vi "Register gRPC Messages.vi"(8 "error in (no error)":errorcluster, 11 "gRPC ID":T1) -> (0 "error out":errorcluster, 3 "gRPC ID Out":T1)   [LabVIEW 2019, in "Generated_server.lvlib"]
uses:
  Generated_server.lvlib
  <vilib>/gRPC/LabVIEW gRPC Library/grpc-lvsupport-release.lvlib
  <vilib>/gRPC/LabVIEW gRPC Library/Server API/typeDefs/Message Metadata.ctl
  <vilib>/gRPC/LabVIEW gRPC Library/Server API/typeDefs/Message Element Type.ctl
  <vilib>/gRPC/LabVIEW gRPC Library/Server API/typeDefs/Message Element Metadata.ctl
  <vilib>/gRPC/LabVIEW gRPC Library/Server API/typeDefs/Enum Metadata.ctl
  <vilib>/gRPC/LabVIEW gRPC Library/Shared/grpcId.ctl
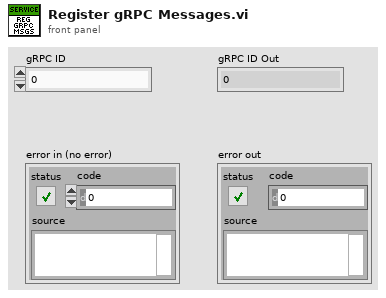
[diagram p1: front panel]
types:
  T1 = typedef "grpc-lvsupport-release.lvlib/grpcId.ctl" = u64
  T2 = typedef "grpc-lvsupport-release.lvlib/Enum Metadata.ctl" = cluster{"Version":i32, "Name":string, "Type Url":string, "Enum Values":string, "Allow Alias":bool}
  T3 = typedef "grpc-lvsupport-release.lvlib/Message Metadata.ctl" = cluster{"Version":i32, "Name":string, "Type Url":string, "Elements":T4[], "Has Oneof":bool}
  T4 = typedef "grpc-lvsupport-release.lvlib/Message Element Metadata.ctl" = cluster{"Field Name":string, "Embedded Message Name":string, "Protobuf Index":i32, "MessageElementType":T5, "Repeated":bool, "Is in Oneof":bool, "Oneof Container Name":string}
  T5 = typedef "grpc-lvsupport-release.lvlib/Message Element Type.ctl" = enum32{"Int32Value", "FloatValue", "DoubleValue", "BoolValue", "StringValue", "MessageValue", "Int64Value", "UInt32Value", "UInt64Value", "EnumValue", "Bytes", "Fixed64", "Fixed32", "SFixed64", "SFixed32", "SInt64", "SInt32"}
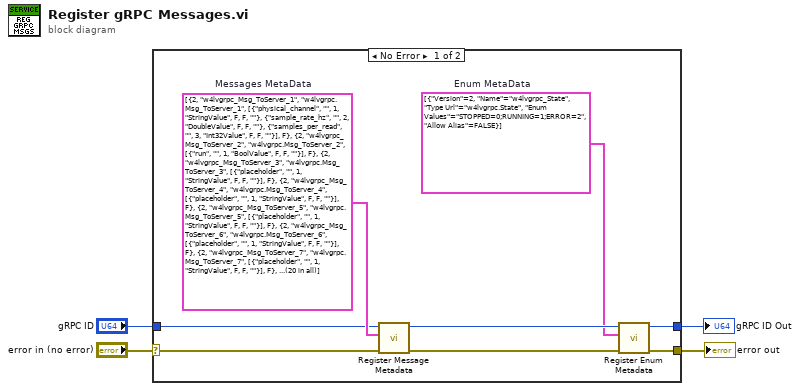
[diagram p0: block diagram]
diagram:
  n1 = case shown="No Error" "error in (no error)" {
    selector: "error in (no error)" -> [w10 w13]
    tunnel: [w9 w12] -> w2
    tunnel: [w6 w13] -> w1
    tunnel: "gRPC ID" -> [w9 w12]
    frame No Error {
      w5 = T2[] [{"Version"=2, "Name"="w4lvgrpc_State", "Type Url"="w4lvgrpc.State", "Enum Values"="STOPPED=0;RUNNING=1;ERROR=2", "Allow Alias"=FALSE}]  # Enum MetaData
      w11 = T3[] [{"Version"=2, "Name"="w4lvgrpc_Msg_ToServer_1", "Type Url"="w4lvgrpc.Msg_ToServer_1", "Elements"=[{"Field Name"="physical_channel", "Embedded Message Name"="", "Protobuf Index"=1, "MessageElementType"=enum."StringValue", "Repeated"=FALSE, "Is in Oneof"=FALSE, "Oneof Container Name"=""}, {"Field Name"="sample_rate_hz", "Embedded Message Name"="", "Protobuf Index"=2, "MessageElementType"=enum."DoubleValue", "Repeated"=FALSE, "Is in Oneof"=FALSE, "Oneof Container Name"=""}, {"Field Name"="samples_per_read", "Embedded Message Name"="", "Protobuf Index"=3, "MessageElementType"=enum."Int32Value", "Repeated"=FALSE, "Is in Oneof"=FALSE, "Oneof Container Name"=""}], "Has Oneof"=FALSE}, {"Version"=2, "Name"="w4lvgrpc_Msg_ToServer_2", "Type Url"="w4lvgrpc.Msg_ToServer_2", "Elements"=[{"Field Name"="run", "Embedded Message Name"="", "Protobuf Index"=1, "MessageElementType"=enum."BoolValue", "Repeated"=FALSE, "Is in Oneof"=FALSE, "Oneof Container Name"=""}], "Has Oneof"=FALSE}, {"Version"=2, "Name"="w4lvgrpc_Msg_ToServer_3", "Type Url"="w4lvgrpc.Msg_ToServer_3", "Elements"=[{"Field Name"="placeholder", "Embedded Message Name"="", "Protobuf Index"=1, "MessageElementType"=enum."StringValue", "Repeated"=FALSE, "Is in Oneof"=FALSE, "Oneof Container Name"=""}], "Has Oneof"=FALSE}, {"Version"=2, "Name"="w4lvgrpc_Msg_ToServer_4", "Type Url"="w4lvgrpc.Msg_ToServer_4", "Elements"=[{"Field Name"="placeholder", "Embedded Message Name"="", "Protobuf Index"=1, "MessageElementType"=enum."StringValue", "Repeated"=FALSE, "Is in Oneof"=FALSE, "Oneof Container Name"=""}], "Has Oneof"=FALSE}, {"Version"=2, "Name"="w4lvgrpc_Msg_ToServer_5", "Type Url"="w4lvgrpc.Msg_ToServer_5", "Elements"=[{"Field Name"="placeholder", "Embedded Message Name"="", "Protobuf Index"=1, "MessageElementType"=enum."StringValue", "Repeated"=FALSE, "Is in Oneof"=FALSE, "Oneof Container Name"=""}], "Has Oneof"=FALSE}, {"Version"=2, "Name"="w4lvgrpc_Msg_ToServer_6", "Type Url"="w4lvgrpc.Msg_ToServer_6", "Elements"=[{"Field Name"="placeholder", "Embedded Message Name"="", "Protobuf Index"=1, "MessageElementType"=enum."StringValue", "Repeated"=FALSE, "Is in Oneof"=FALSE, "Oneof Container Name"=""}], "Has Oneof"=FALSE}, {"Version"=2, "Name"="w4lvgrpc_Msg_ToServer_7", "Type Url"="w4lvgrpc.Msg_ToServer_7", "Elements"=[{"Field Name"="placeholder", "Embedded Message Name"="", "Protobuf Index"=1, "MessageElementType"=enum."StringValue", "Repeated"=FALSE, "Is in Oneof"=FALSE, "Oneof Container Name"=""}], "Has Oneof"=FALSE}, {"Version"=2, "Name"="w4lvgrpc_Msg_ToServer_8", "Type Url"="w4lvgrpc.Msg_ToServer_8", "Elements"=[{"Field Name"="placeholder", "Embedded Message Name"="", "Protobuf Index"=1, "MessageElementType"=enum."StringValue", "Repeated"=FALSE, "Is in Oneof"=FALSE, "Oneof Container Name"=""}], "Has Oneof"=FALSE}, {"Version"=2, "Name"="w4lvgrpc_Msg_ToServer_9", "Type Url"="w4lvgrpc.Msg_ToServer_9", "Elements"=[{"Field Name"="placeholder", "Embedded Message Name"="", "Protobuf Index"=1, "MessageElementType"=enum."StringValue", "Repeated"=FALSE, "Is in Oneof"=FALSE, "Oneof Container Name"=""}], "Has Oneof"=FALSE}, {"Version"=2, "Name"="w4lvgrpc_Msg_ToClient_1", "Type Url"="w4lvgrpc.Msg_ToClient_1", "Elements"=[{"Field Name"="device", "Embedded Message Name"="", "Protobuf Index"=1, "MessageElementType"=enum."StringValue", "Repeated"=FALSE, "Is in Oneof"=FALSE, "Oneof Container Name"=""}, {"Field Name"="product_type", "Embedded Message Name"="", "Protobuf Index"=2, "MessageElementType"=enum."StringValue", "Repeated"=FALSE, "Is in Oneof"=FALSE, "Oneof Container Name"=""}], "Has Oneof"=FALSE}, {"Version"=2, "Name"="w4lvgrpc_Msg_ToClient_2", "Type Url"="w4lvgrpc.Msg_ToClient_2", "Elements"=[{"Field Name"="y", "Embedded Message Name"="", "Protobuf Index"=1, "MessageElementType"=enum."DoubleValue", "Repeated"=TRUE, "Is in Oneof"=FALSE, "Oneof Container Name"=""}, {"Field Name"="dt", "Embedded Message Name"="", "Protobuf Index"=2, "MessageElementType"=enum."DoubleValue", "Repeated"=FALSE, "Is in Oneof"=FALSE, "Oneof Container Name"=""}, {"Field Name"="t0", "Embedded Message Name"="", "Protobuf Index"=3, "MessageElementType"=enum."DoubleValue", "Repeated"=FALSE, "Is in Oneof"=FALSE, "Oneof Container Name"=""}, {"Field Name"="label", "Embedded Message Name"="", "Protobuf Index"=4, "MessageElementType"=enum."StringValue", "Repeated"=FALSE, "Is in Oneof"=FALSE, "Oneof Container Name"=""}, {"Field Name"="acquisitions", "Embedded Message Name"="", "Protobuf Index"=5, "MessageElementType"=enum."Int32Value", "Repeated"=FALSE, "Is in Oneof"=FALSE, "Oneof Container Name"=""}], "Has Oneof"=FALSE}, {"Version"=2, "Name"="w4lvgrpc_Msg_ToClient_3", "Type Url"="w4lvgrpc.Msg_ToClient_3", "Elements"=[{"Field Name"="state", "Embedded Message Name"="w4lvgrpc_State", "Protobuf Index"=1, "MessageElementType"=enum."EnumValue", "Repeated"=FALSE, "Is in Oneof"=FALSE, "Oneof Container Name"=""}], "Has Oneof"=FALSE}, {"Version"=2, "Name"="w4lvgrpc_Msg_ToClient_4", "Type Url"="w4lvgrpc.Msg_ToClient_4", "Elements"=[{"Field Name"="placeholder", "Embedded Message Name"="", "Protobuf Index"=1, "MessageElementType"=enum."StringValue", "Repeated"=FALSE, "Is in Oneof"=FALSE, "Oneof Container Name"=""}], "Has Oneof"=FALSE}, {"Version"=2, "Name"="w4lvgrpc_Msg_ToClient_5", "Type Url"="w4lvgrpc.Msg_ToClient_5", "Elements"=[{"Field Name"="placeholder", "Embedded Message Name"="", "Protobuf Index"=1, "MessageElementType"=enum."StringValue", "Repeated"=FALSE, "Is in Oneof"=FALSE, "Oneof Container Name"=""}], "Has Oneof"=FALSE}, {"Version"=2, "Name"="w4lvgrpc_Msg_ToClient_6", "Type Url"="w4lvgrpc.Msg_ToClient_6", "Elements"=[{"Field Name"="placeholder", "Embedded Message Name"="", "Protobuf Index"=1, "MessageElementType"=enum."StringValue", "Repeated"=FALSE, "Is in Oneof"=FALSE, "Oneof Container Name"=""}], "Has Oneof"=FALSE}, {"Version"=2, "Name"="w4lvgrpc_Msg_ToClient_7", "Type Url"="w4lvgrpc.Msg_ToClient_7", "Elements"=[{"Field Name"="placeholder", "Embedded Message Name"="", "Protobuf Index"=1, "MessageElementType"=enum."StringValue", "Repeated"=FALSE, "Is in Oneof"=FALSE, "Oneof Container Name"=""}], "Has Oneof"=FALSE}, {"Version"=2, "Name"="w4lvgrpc_Msg_ToClient_8", "Type Url"="w4lvgrpc.Msg_ToClient_8", "Elements"=[{"Field Name"="placeholder", "Embedded Message Name"="", "Protobuf Index"=1, "MessageElementType"=enum."StringValue", "Repeated"=FALSE, "Is in Oneof"=FALSE, "Oneof Container Name"=""}], "Has Oneof"=FALSE}, {"Version"=2, "Name"="w4lvgrpc_Msg_ToClient_9", "Type Url"="w4lvgrpc.Msg_ToClient_9", "Elements"=[{"Field Name"="placeholder", "Embedded Message Name"="", "Protobuf Index"=1, "MessageElementType"=enum."StringValue", "Repeated"=FALSE, "Is in Oneof"=FALSE, "Oneof Container Name"=""}], "Has Oneof"=FALSE}, {"Version"=2, "Name"="w4lvgrpc_ToServer", "Type Url"="w4lvgrpc.ToServer", "Elements"=[{"Field Name"="selected_index", "Embedded Message Name"="", "Protobuf Index"=-1, "MessageElementType"=enum."Int32Value", "Repeated"=FALSE, "Is in Oneof"=TRUE, "Oneof Container Name"="w4lvgrpc_ToServer_payload"}, {"Field Name"="msg_1", "Embedded Message Name"="w4lvgrpc_Msg_ToServer_1", "Protobuf Index"=1, "MessageElementType"=enum."MessageValue", "Repeated"=FALSE, "Is in Oneof"=TRUE, "Oneof Container Name"="w4lvgrpc_ToServer_payload"}, {"Field Name"="msg_2", "Embedded Message Name"="w4lvgrpc_Msg_ToServer_2", "Protobuf Index"=2, "MessageElementType"=enum."MessageValue", "Repeated"=FALSE, "Is in Oneof"=TRUE, "Oneof Container Name"="w4lvgrpc_ToServer_payload"}, {"Field Name"="msg_3", "Embedded Message Name"="w4lvgrpc_Msg_ToServer_3", "Protobuf Index"=3, "MessageElementType"=enum."MessageValue", "Repeated"=FALSE, "Is in Oneof"=TRUE, "Oneof Container Name"="w4lvgrpc_ToServer_payload"}, {"Field Name"="msg_4", "Embedded Message Name"="w4lvgrpc_Msg_ToServer_4", "Protobuf Index"=4, "MessageElementType"=enum."MessageValue", "Repeated"=FALSE, "Is in Oneof"=TRUE, "Oneof Container Name"="w4lvgrpc_ToServer_payload"}, {"Field Name"="msg_5", "Embedded Message Name"="w4lvgrpc_Msg_ToServer_5", "Protobuf Index"=5, "MessageElementType"=enum."MessageValue", "Repeated"=FALSE, "Is in Oneof"=TRUE, "Oneof Container Name"="w4lvgrpc_ToServer_payload"}, {"Field Name"="msg_6", "Embedded Message Name"="w4lvgrpc_Msg_ToServer_6", "Protobuf Index"=6, "MessageElementType"=enum."MessageValue", "Repeated"=FALSE, "Is in Oneof"=TRUE, "Oneof Container Name"="w4lvgrpc_ToServer_payload"}, {"Field Name"="msg_7", "Embedded Message Name"="w4lvgrpc_Msg_ToServer_7", "Protobuf Index"=7, "MessageElementType"=enum."MessageValue", "Repeated"=FALSE, "Is in Oneof"=TRUE, "Oneof Container Name"="w4lvgrpc_ToServer_payload"}, {"Field Name"="msg_8", "Embedded Message Name"="w4lvgrpc_Msg_ToServer_8", "Protobuf Index"=8, "MessageElementType"=enum."MessageValue", "Repeated"=FALSE, "Is in Oneof"=TRUE, "Oneof Container Name"="w4lvgrpc_ToServer_payload"}, {"Field Name"="msg_9", "Embedded Message Name"="w4lvgrpc_Msg_ToServer_9", "Protobuf Index"=9, "MessageElementType"=enum."MessageValue", "Repeated"=FALSE, "Is in Oneof"=TRUE, "Oneof Container Name"="w4lvgrpc_ToServer_payload"}], "Has Oneof"=TRUE}, {"Version"=2, "Name"="w4lvgrpc_ToClient", "Type Url"="w4lvgrpc.ToClient", "Elements"=[{"Field Name"="selected_index", "Embedded Message Name"="", "Protobuf Index"=-1, "MessageElementType"=enum."Int32Value", "Repeated"=FALSE, "Is in Oneof"=TRUE, "Oneof Container Name"="w4lvgrpc_ToClient_payload"}, {"Field Name"="msg_1", "Embedded Message Name"="w4lvgrpc_Msg_ToClient_1", "Protobuf Index"=1, "MessageElementType"=enum."MessageValue", "Repeated"=FALSE, "Is in Oneof"=TRUE, "Oneof Container Name"="w4lvgrpc_ToClient_payload"}, {"Field Name"="msg_2", "Embedded Message Name"="w4lvgrpc_Msg_ToClient_2", "Protobuf Index"=2, "MessageElementType"=enum."MessageValue", "Repeated"=FALSE, "Is in Oneof"=TRUE, "Oneof Container Name"="w4lvgrpc_ToClient_payload"}, {"Field Name"="msg_3", "Embedded Message Name"="w4lvgrpc_Msg_ToClient_3", "Protobuf Index"=3, "MessageElementType"=enum."MessageValue", "Repeated"=FALSE, "Is in Oneof"=TRUE, "Oneof Container Name"="w4lvgrpc_ToClient_payload"}, {"Field Name"="msg_4", "Embedded Message Name"="w4lvgrpc_Msg_ToClient_4", "Protobuf Index"=4, "MessageElementType"=enum."MessageValue", "Repeated"=FALSE, "Is in Oneof"=TRUE, "Oneof Container Name"="w4lvgrpc_ToClient_payload"}, {"Field Name"="msg_5", "Embedded Message Name"="w4lvgrpc_Msg_ToClient_5", "Protobuf Index"=5, "MessageElementType"=enum."MessageValue", "Repeated"=FALSE, "Is in Oneof"=TRUE, "Oneof Container Name"="w4lvgrpc_ToClient_payload"}, {"Field Name"="msg_6", "Embedded Message Name"="w4lvgrpc_Msg_ToClient_6", "Protobuf Index"=6, "MessageElementType"=enum."MessageValue", "Repeated"=FALSE, "Is in Oneof"=TRUE, "Oneof Container Name"="w4lvgrpc_ToClient_payload"}, {"Field Name"="msg_7", "Embedded Message Name"="w4lvgrpc_Msg_ToClient_7", "Protobuf Index"=7, "MessageElementType"=enum."MessageValue", "Repeated"=FALSE, "Is in Oneof"=TRUE, "Oneof Container Name"="w4lvgrpc_ToClient_payload"}, {"Field Name"="msg_8", "Embedded Message Name"="w4lvgrpc_Msg_ToClient_8", "Protobuf Index"=8, "MessageElementType"=enum."MessageValue", "Repeated"=FALSE, "Is in Oneof"=TRUE, "Oneof Container Name"="w4lvgrpc_ToClient_payload"}, {"Field Name"="msg_9", "Embedded Message Name"="w4lvgrpc_Msg_ToClient_9", "Protobuf Index"=9, "MessageElementType"=enum."MessageValue", "Repeated"=FALSE, "Is in Oneof"=TRUE, "Oneof Container Name"="w4lvgrpc_ToClient_payload"}], "Has Oneof"=TRUE}]  # Messages MetaData
      n2 = call <vilib>:"Register Message Metadata.vi"("error in"=w10, "Messages"=w11, "gRPCid in"=w9) -> ("error out"=w7:errorcluster, "gRPCid out"=w8:T1)  [unwired: 7 in]
      n3 = call <vilib>:"Register Enum Metadata.vi"("error in"=w7, "Enum Metadata"=w5, "gRPCid in"=w8) -> ("error out"=w6:errorcluster)  [unwired: 7 in, 1 out]
    }
    frame Error {
    }
  }
  "error out" <- w1
  "gRPC ID Out" <- w2
